vi "Tree Selection FGV.vi"(7 "Action":T8, 8 "error in (no error)":errorcluster, 9 "Mouse down data":T7, 10 "States":bool[](array[boolean]), 11 "Listbox or Tree":refnum<vi>) -> (0 "error out":errorcluster, 3 "read data":T1)   [LabVIEW 2020, in "UI_ItemSelect_OpenSource.lvlib"]
uses:
  UI_ItemSelect_OpenSource.lvlib
  item select action.ctl
  item select mouse down data.ctl
  Tree item select loop data.ctl
  Item select ref type.ctl
  Tree item loop data.ctl
  Tree item selection indices.ctl
  checkbox state.ctl
  item select tree lock states.ctl
  <userlib>/Blue Origin/DeferPanelUpdates_OpenSource/SubVIs/defer panel updates Controlref step1.vi
  <userlib>/Blue Origin/DeferPanelUpdates_OpenSource/SubVIs/defer panel updates step2.vi
  <vilib>/Utility/error.llb/Error Cluster From Error Code.vi
  <vilib>/ErrorRing/Error Ring.xnode
  <userlib>/Blue Origin/DeferPanelUpdates_OpenSource/Defer Panel Updates OpenSource.lvlib
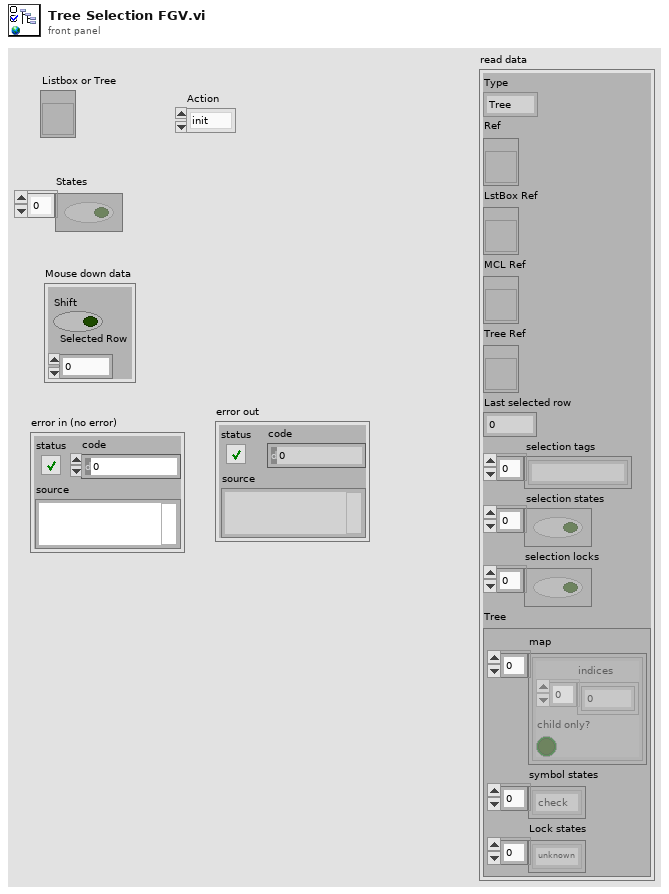
[diagram p1: front panel]
types:
  T1 = typedef "UI_ItemSelect_OpenSource.lvlib/Tree item select loop data.ctl" = cluster{"Type":T2, "Ref":refnum<vi>, "LstBox Ref":refnum<vi>, "MCL Ref":refnum<vi>, "Tree Ref":refnum<vi>, "Last selected row":i32, "selection tags":string[], "selection states":bool[], "selection locks":bool[], "Tree":T3}
  T2 = typedef "UI_ItemSelect_OpenSource.lvlib/Item select ref type.ctl" = enum16{"Tree", "MCL", "ListBox"}
  T3 = typedef "UI_ItemSelect_OpenSource.lvlib/Tree item loop data.ctl" = cluster{"map":T4[], "symbol states":T5[], "Lock states":T6[]}
  T4 = typedef "UI_ItemSelect_OpenSource.lvlib/Tree item selection indices.ctl" = cluster{"indices":i32[], "child only?":bool}
  T5 = typedef "UI_ItemSelect_OpenSource.lvlib/checkbox state.ctl" = enum16{"unknown", "check", "some", "no check"}
  T6 = typedef "UI_ItemSelect_OpenSource.lvlib/item select tree lock states.ctl" = enum16{"unknown", "locked", "unlocked"}
  T7 = typedef "UI_ItemSelect_OpenSource.lvlib/item select mouse down data.ctl" = cluster{"Shift":bool, "Selected Row":i32}
  T8 = typedef "UI_ItemSelect_OpenSource.lvlib/item select action.ctl" = enum16{"init", "read", "write states", "write locks", "mouse down", "delete", "select all", "select none", "invert selection"}
  T9 = typedef "Defer Panel Updates OpenSource.lvlib/defer panel updates data.ctl" = cluster{"Owning VI":refnum<vi>, "Front Panel":refnum<vi>, "performed?":bool}
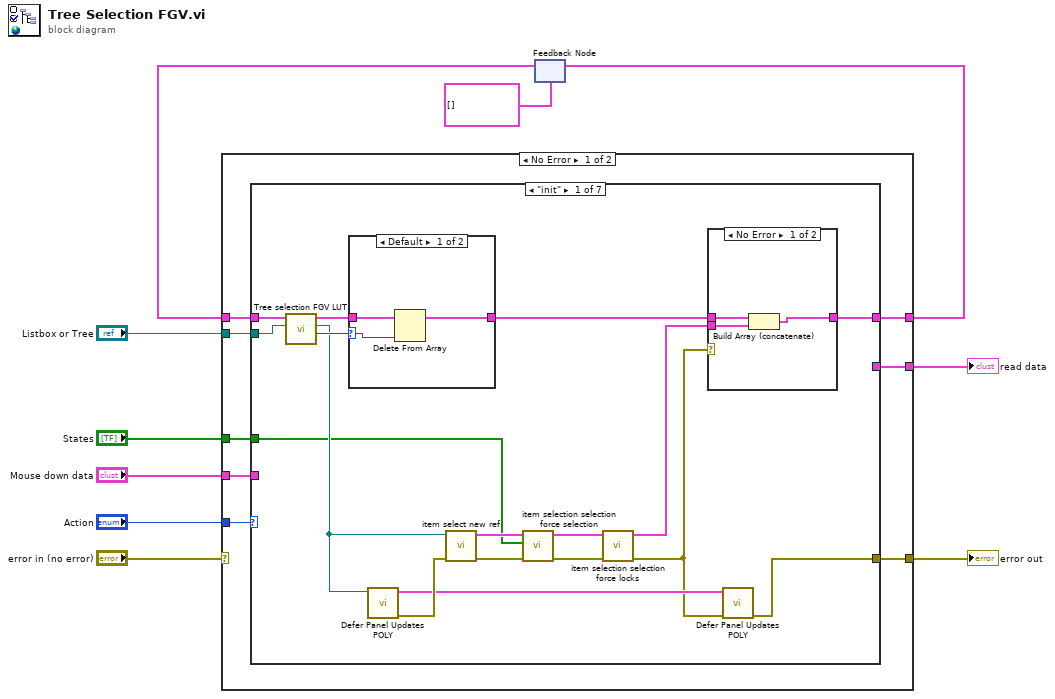
[diagram p0: block diagram]
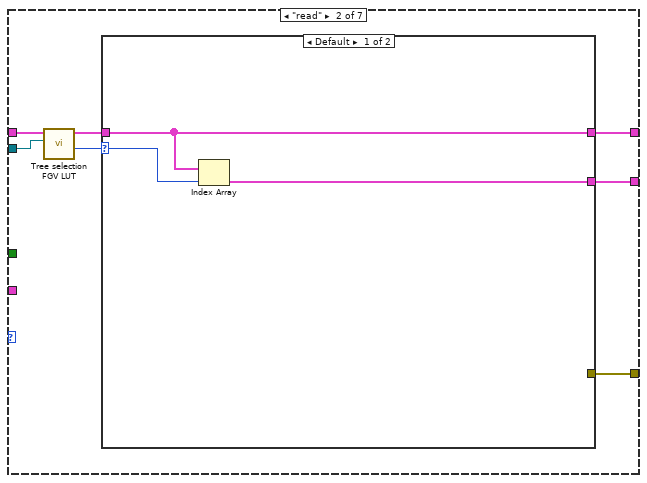
[diagram p4: hidden frame]
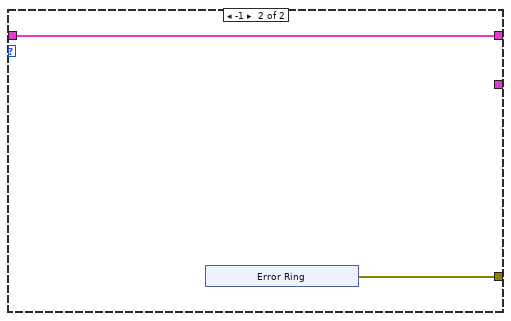
[diagram p5: hidden frame]
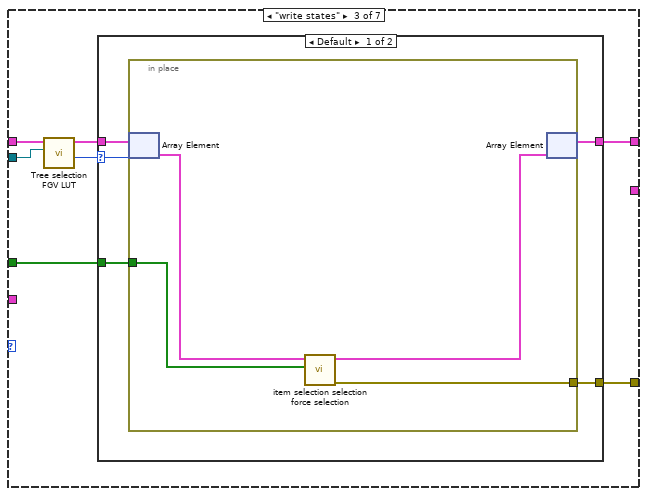
[diagram p6: hidden frame]
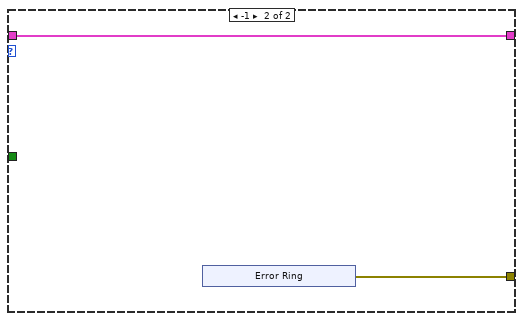
[diagram p7: hidden frame]
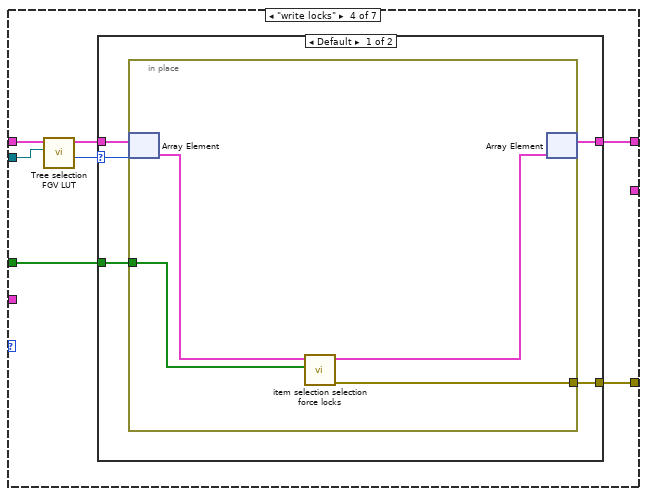
[diagram p8: hidden frame]
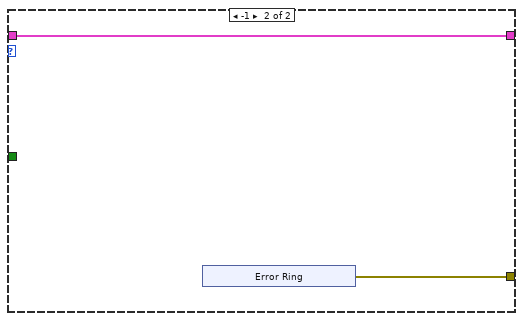
[diagram p9: hidden frame]
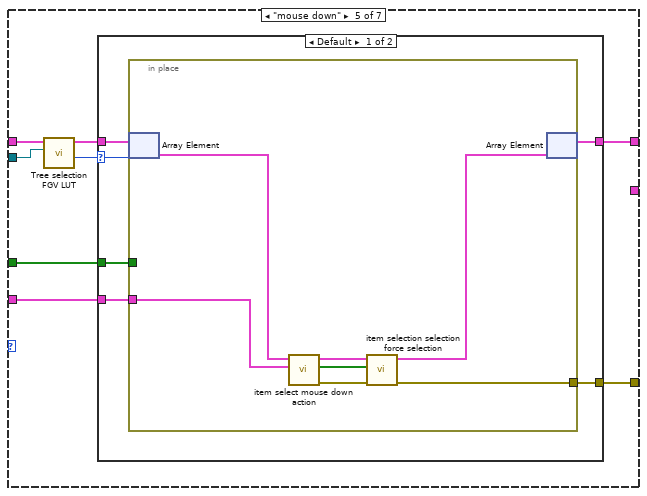
[diagram p10: hidden frame]
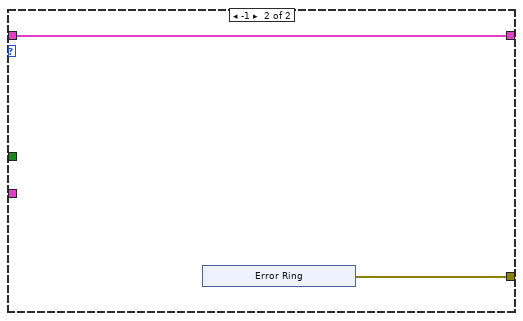
[diagram p11: hidden frame]
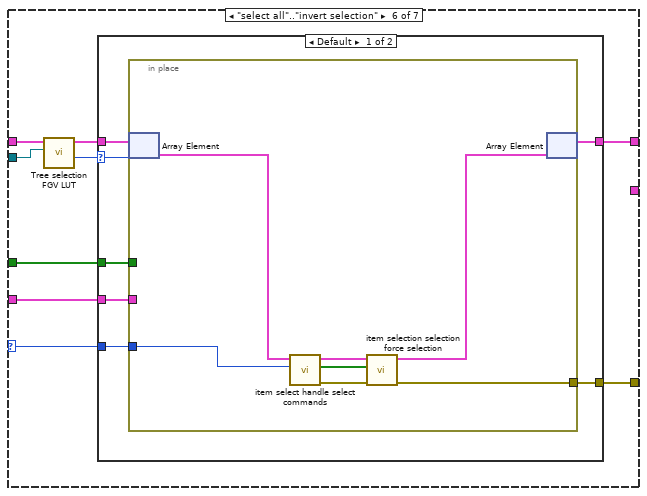
[diagram p12: hidden frame]
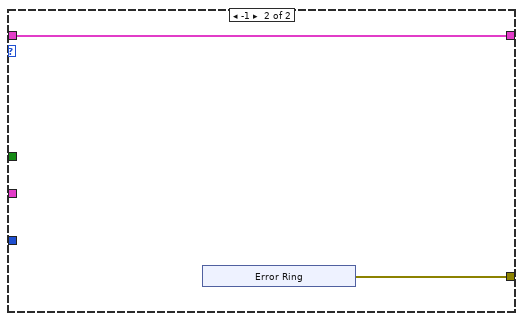
[diagram p13: hidden frame]
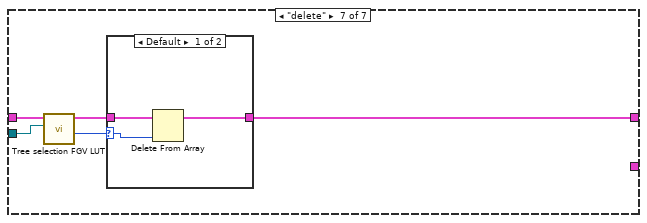
[diagram p14: hidden frame]
diagram:
  n1 = feedback #1(T1[] [] ("Data")) -> (w10:T1[])
  n2 = case shown="No Error" "error in (no error)" {
    selector: "error in (no error)" -> [_ w175]
    tunnel: w10 -> [w18 w174]
    tunnel: "States" -> [w17 _]
    tunnel: [w16 w174] -> w8
    tunnel: "Listbox or Tree" -> [w15 _]
    tunnel: "Action" -> [w14 _]
    tunnel: [w13 w175] -> w3
    tunnel: "Mouse down data" -> [w12 _]
    tunnel: [w11 _] -> w1
    frame No Error {
      n3 = case shown="\"init\"" w14 {
        selector: w14 -> [_ _ _ _ _ w135 _]
        tunnel: w18 -> [w35 w50 w67 w90 w114 w143 w169]
        tunnel: w15 -> [w32 w47 w66 w89 w113 w142 w166]
        tunnel: w17 -> [w19 _ w61 w84 w108 w137 _]
        tunnel: [w28 w46 w62 w85 w109 w138 w165] -> w16
        tunnel: [w20 w45 w64 w87 w111 w140 _] -> w13
        tunnel: w12 -> [_ _ _ _ w107 w136 _]
        tunnel: [_ w44 _ _ _ _ _] -> w11
        frame "init" {
          n4 = call "Tree selection FGV LUT.vi"("Ref"=w32, "Loop data"=w35) -> ("Index"=w33:i32, "Ref (dup)"=w23:refnum<vi>, "Loop data"=w34:T1[])  [unwired: 7 in]
          n5 = case shown="Default" w33 {
            selector: w33 -> [w41 _]
            tunnel: w34 -> [w42 w43]
            tunnel: [w40 w43] -> w29
            frame Default {
              n6 = Delete From Array(array=w42, index=w41) -> (array with subset deleted=w40:T1[])  [unwired: 1 in, 1 out]
            }
            frame -1 {
            }
          }
          n7 = call-poly <userlib>:"Defer Panel Updates POLY.vi"("control reference"=w23) -> ("error out"=w24:errorcluster, "Refs"=w22:T9)  [unwired: 9 in]
          n8 = call "item select new ref.vi"("error in (no error)"=w24, "Listbox or Tree"=w23) -> ("error out"=w30:errorcluster, "Loop data"=w31:T1)  [unwired: 8 in]
          n9 = call "item selection selection force selection.vi"("error in (no error)"=w30, "Selection States"=w19, "Loop data"=w31) -> ("error out"=w26:errorcluster, "Loop data"=w27:T1)  [unwired: 7 in]
          n10 = call "item selection selection force locks.vi"("error in (no error)"=w26, "Loop data"=w27) -> ("error out"=w21:errorcluster, "Loop data"=w25:T1)  [unwired: 8 in]
          n11 = case shown="No Error" w21 {
            tunnel: w29 -> [w38 w39]
            tunnel: [w37 w39] -> w28
            tunnel: w25 -> [w36 _]
            frame No Error {
              n12 = Build Array (concatenate)(w38, w36) -> (w37:T1[])
            }
            frame Error {
            }
          }
          n13 = call-poly <userlib>:"Defer Panel Updates POLY.vi"("error in (no error)"=w21, "Refs"=w22) -> ("error out"=w20:errorcluster)  [unwired: 9 in]
        }
        frame "read" {
          n14 = call "Tree selection FGV LUT.vi"("Ref"=w47, "Loop data"=w50) -> ("Index"=w48:i32, "Loop data"=w49:T1[])  [unwired: 7 in, 1 out]
          n15 = case shown="Default" w48 {
            selector: w48 -> [w52 _]
            tunnel: w49 -> [w53 w55]
            tunnel: [w53 w55] -> w46
            tunnel: [_ w54] -> w45
            tunnel: [w51 _] -> w44
            frame Default {
              n16 = Index Array(array=w53, index=w52) -> (element=w51:T1)
            }
            frame -1 {
              n17 = xnode "Error Ring"() -> ("error out"=w54:errorcluster)
            }
          }
        }
        frame "write states" {
          n18 = call "Tree selection FGV LUT.vi"("Ref"=w66, "Loop data"=w67) -> ("Index"=w65:i32, "Loop data"=w63:T1[])  [unwired: 7 in, 1 out]
          n19 = case shown="Default" w65 {
            selector: w65 -> [w70 _]
            tunnel: [w72 w78] -> w64
            tunnel: w63 -> [w71 w77]
            tunnel: [w69 w77] -> w62
            tunnel: w61 -> [w68 _]
            frame Default {
              n20 = in-place {
                in-place-border: [w76] -> w72
                in-place-border: w68 -> [w74]
                n21 = in-place-array #2(w71, w70) -> (w75:T1)
                n22 = call "item selection selection force selection.vi"("Selection States"=w74, "Loop data"=w75) -> ("error out"=w76:errorcluster, "Loop data"=w73:T1)  [unwired: 8 in]
                n23 = in-place-array #2(w73) -> (w69:T1[])  [unwired: 1 out]
              }
            }
            frame -1 {
              n24 = xnode "Error Ring"() -> ("error out"=w78:errorcluster)
            }
          }
        }
        frame "write locks" {
          n25 = call "Tree selection FGV LUT.vi"("Ref"=w89, "Loop data"=w90) -> ("Index"=w88:i32, "Loop data"=w86:T1[])  [unwired: 7 in, 1 out]
          n26 = case shown="Default" w88 {
            selector: w88 -> [w93 _]
            tunnel: [w95 w101] -> w87
            tunnel: w86 -> [w94 w100]
            tunnel: [w92 w100] -> w85
            tunnel: w84 -> [w91 _]
            frame Default {
              n27 = in-place {
                in-place-border: [w96] -> w95
                in-place-border: w91 -> [w98]
                n28 = in-place-array #3(w94, w93) -> (w99:T1)
                n29 = call "item selection selection force locks.vi"("Lock States"=w98, "Loop data"=w99) -> ("error out"=w96:errorcluster, "Loop data"=w97:T1)  [unwired: 8 in]
                n30 = in-place-array #3(w97) -> (w92:T1[])  [unwired: 1 out]
              }
            }
            frame -1 {
              n31 = xnode "Error Ring"() -> ("error out"=w101:errorcluster)
            }
          }
        }
        frame "mouse down" {
          n32 = call "Tree selection FGV LUT.vi"("Ref"=w113, "Loop data"=w114) -> ("Index"=w112:i32, "Loop data"=w110:T1[])  [unwired: 7 in, 1 out]
          n33 = case shown="Default" w112 {
            selector: w112 -> [w118 _]
            tunnel: [w120 w129] -> w111
            tunnel: w110 -> [w119 w128]
            tunnel: [w117 w128] -> w109
            tunnel: w108 -> [w116 _]
            tunnel: w107 -> [w115 _]
            frame Default {
              n34 = in-place {
                in-place-border: [w127] -> w120
                in-place-border: w116 -> [_]
                in-place-border: w115 -> [w121]
                n35 = in-place-array #4(w119, w118) -> (w122:T1)
                n36 = call "item select mouse down action.vi"("Mouse down data"=w121, "Loop data"=w122) -> ("error out"=w124:errorcluster, "New Selection states"=w123:bool[], "Loop data"=w125:T1)  [unwired: 7 in]
                n37 = call "item selection selection force selection.vi"("error in (no error)"=w124, "Selection States"=w123, "Loop data"=w125) -> ("error out"=w127:errorcluster, "Loop data"=w126:T1)  [unwired: 7 in]
                n38 = in-place-array #4(w126) -> (w117:T1[])  [unwired: 1 out]
              }
            }
            frame -1 {
              n39 = xnode "Error Ring"() -> ("error out"=w129:errorcluster)
            }
          }
        }
        frame "select all".."invert selection" {
          n40 = call "Tree selection FGV LUT.vi"("Ref"=w142, "Loop data"=w143) -> ("Index"=w141:i32, "Loop data"=w139:T1[])  [unwired: 7 in, 1 out]
          n41 = case shown="Default" w141 {
            selector: w141 -> [w148 _]
            tunnel: [w150 w159] -> w140
            tunnel: w139 -> [w149 w158]
            tunnel: [w147 w158] -> w138
            tunnel: w137 -> [w146 _]
            tunnel: w136 -> [w145 _]
            tunnel: w135 -> [w144 _]
            frame Default {
              n42 = in-place {
                in-place-border: [w157] -> w150
                in-place-border: w146 -> [_]
                in-place-border: w145 -> [_]
                in-place-border: w144 -> [w151]
                n43 = in-place-array #5(w149, w148) -> (w155:T1)
                n44 = call "item select handle select commands.vi"("Action"=w151, "Loop data"=w155) -> ("error out"=w152:errorcluster, "New Selection states"=w153:bool[], "Loop data"=w154:T1)  [unwired: 7 in]
                n45 = call "item selection selection force selection.vi"("error in (no error)"=w152, "Selection States"=w153, "Loop data"=w154) -> ("error out"=w157:errorcluster, "Loop data"=w156:T1)  [unwired: 7 in]
                n46 = in-place-array #5(w156) -> (w147:T1[])  [unwired: 1 out]
              }
            }
            frame -1 {
              n47 = xnode "Error Ring"() -> ("error out"=w159:errorcluster)
            }
          }
        }
        frame "delete" {
          n48 = call "Tree selection FGV LUT.vi"("Ref"=w166, "Loop data"=w169) -> ("Index"=w167:i32, "Loop data"=w168:T1[])  [unwired: 7 in, 1 out]
          n49 = case shown="Default" w167 {
            selector: w167 -> [w171 _]
            tunnel: w168 -> [w172 w173]
            tunnel: [w170 w173] -> w165
            frame Default {
              n50 = Delete From Array(array=w172, index=w171) -> (array with subset deleted=w170:T1[])  [unwired: 1 in, 1 out]
            }
            frame -1 {
            }
          }
        }
      }
    }
    frame Error {
    }
  }
  "error out" <- w3
  "read data" <- w1
  n51 = feedback-in #1(w8) -> ()
